vi "Write G08 Specific.vi"(8 "error in (no error)":errorcluster, 9 "Output Offset":u32, 10 "Pulse Width (µs)":dbl=0.005 min=0.0 max=8947840.0 format="%.6f", 11 "BME_DG_G08_Chnl in":refnum<class "BME_DG_G08_Chnl.lvclass">) -> (0 "error out":errorcluster, 3 "BME_DG_G08_Chnl out":refnum<class "BME_DG_G08_Chnl.lvclass">)   [LabVIEW 2009, in "POLARIS BME DG.lvlib" / "BME_DG_G08_Chnl.lvclass"]
uses:
  BME_DG_G08_Chnl.lvclass
  BME_DG_G08_Chnl.lvclass/BME_DG_G08_Chnl.ctl
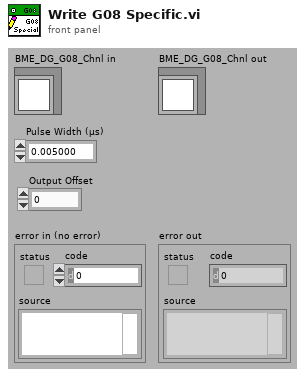
[diagram p1: front panel]
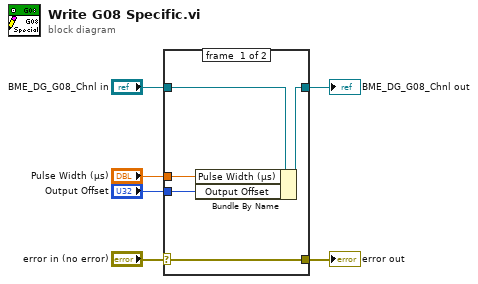
[diagram p0: block diagram]
diagram:
  n1 = case shown="No Error" "error in (no error)" {
    selector: "error in (no error)" -> [w11 w12]
    tunnel: [w11 w12] -> w5
    tunnel: [w9 w13] -> w3
    tunnel: "BME_DG_G08_Chnl in" -> [w10 w13]
    tunnel: "Pulse Width (µs)" -> [w8 _]
    tunnel: "Output Offset" -> [w7 _]
    frame #0 {
      n2 = Bundle By Name(cluster=w10, "Pulse Width (µs)"=w8, "Output Offset"=w7) -> (w9:refnum<class "BME_DG_G08_Chnl.lvclass">)
    }
    frame #1 {
    }
  }
  "error out" <- w5
  "BME_DG_G08_Chnl out" <- w3
